vi "LHF.DB.Mongo.Collection.EnsureIndex.vi"(8 "error in (no error)":errorcluster, 9 "value":variant, 10 "Collection":string, 11 "LHF.DB.Mongo in":refnum<class "LHF.DB.Mongo.lvclass">) -> (0 "error out":errorcluster, 3 "LHF.DB.Mongo out":refnum<class "LHF.DB.Mongo.lvclass">)   [LabVIEW 2013, in "LHF.DB.Mongo.lvclass"]
doc: "Creates an index in collection. Variable name, type & content will be used."
uses:
  LHF.DB.Mongo.lvclass
  C:/Users/Ricardo/Desktop/Projetos/LabVIEW-MongoDB/src/Driver/MongoDB.Driver.dll
  LabVIEW-MongoDB/src/Driver/MongoDB.Driver.dll
  <vilib>/Utility/VariantDataType/VariantType.lvlib
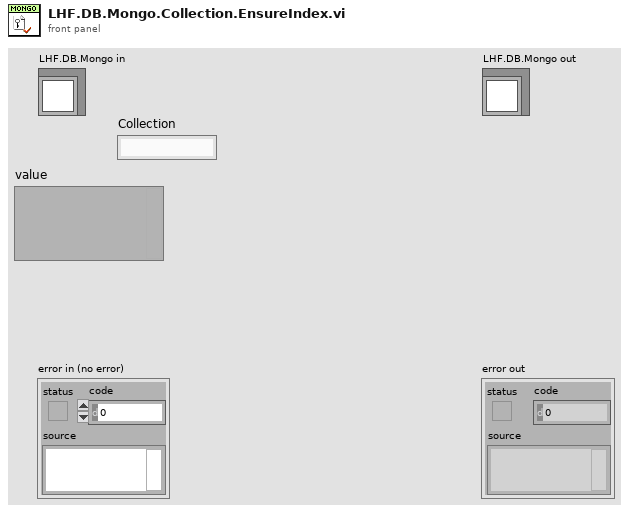
[diagram p1: front panel]
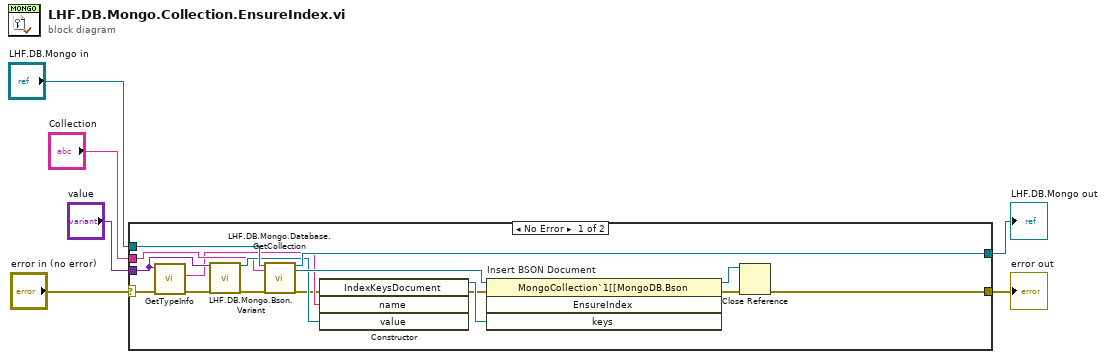
[diagram p0: block diagram]
diagram:
  n1 = case shown="No Error" "error in (no error)" {
    selector: "error in (no error)" -> [w10 w24]
    tunnel: [w7 w24] -> w5
    tunnel: [w20 w23] -> w3
    tunnel: "LHF.DB.Mongo in" -> [w21 w23]
    tunnel: "value" -> [w13 _]
    tunnel: "Collection" -> [w15 _]
    frame No Error {
      n2 = call <vilib>:"GetTypeInfo.vi"("error in (no error)"=w10, "Variant"=w13) -> ("error out"=w11:errorcluster, "Name"=w12:string)  [unwired: 5 in, 3 out]
      n3 = call "LHF.DB.Mongo.Bson.Variant.vi"("Variant"=w13, "error IO"=w11) -> ("BsonValue"=w18:refnum<k24>, "error IO 2"=w9:errorcluster)  [unwired: 16 in]
      n4 = call "LHF.DB.Mongo.Database.GetCollection.vi"("LHF.DB.Mongo in"=w21, "collectionName"=w15, "error in (no error)"=w9) -> ("LHF.DB.Mongo in"=w20:refnum<class "LHF.DB.Mongo.lvclass">, "MongoCollection"=w19:refnum<k24>, "error out"=w8:errorcluster)  [unwired: 14 in]
      n5 = constructor class="IndexKeysDocument"(error in=w8, "name"=w12, "value"=w18) -> (reference out=w22:refnum<k24>, error out=w17:errorcluster)  [unwired: 2 in, 3 out]
      n6 = invoke on="Insert BSON Document" class="MongoCollection`1[[MongoDB.Bson" method="EnsureIndex"(reference=w19, error in=w17, "keys"=w22) -> (reference out=w14:refnum<k24>, error out=w16:errorcluster)  [unwired: 1 in, 2 out]
      n7 = Close Reference(reference=w14, error in (no error)=w16) -> (error out=w7:errorcluster)
    }
    frame Error {
    }
  }
  "error out" <- w5
  "LHF.DB.Mongo out" <- w3
